vi "UpdateField.vi"   [LabVIEW 2025]
uses:
  ServerGlobalVariables.vi
types:
  T1 = typedef "FieldCell.ctl" = cluster{"Troops":u32, "Owner":i32, "Terrain":T2}
  T2 = typedef "TerrainEnum.ctl" = enum16{"Plain", "Mountain", "City", "General"}
  T3 = map{u32, cluster{"Name":string, "Team":u8, "Ready":bool, "Host":bool, "Alive":bool, "Color":u32, "Lands":set{cluster{"Row":u32, "Column":u32}}, "Army":u32}}
  T4 = cluster{"Name":string, "Team":u8, "Ready":bool, "Host":bool, "Alive":bool, "Color":u32, "Lands":set{cluster{"Row":u32, "Column":u32}}, "Army":u32}
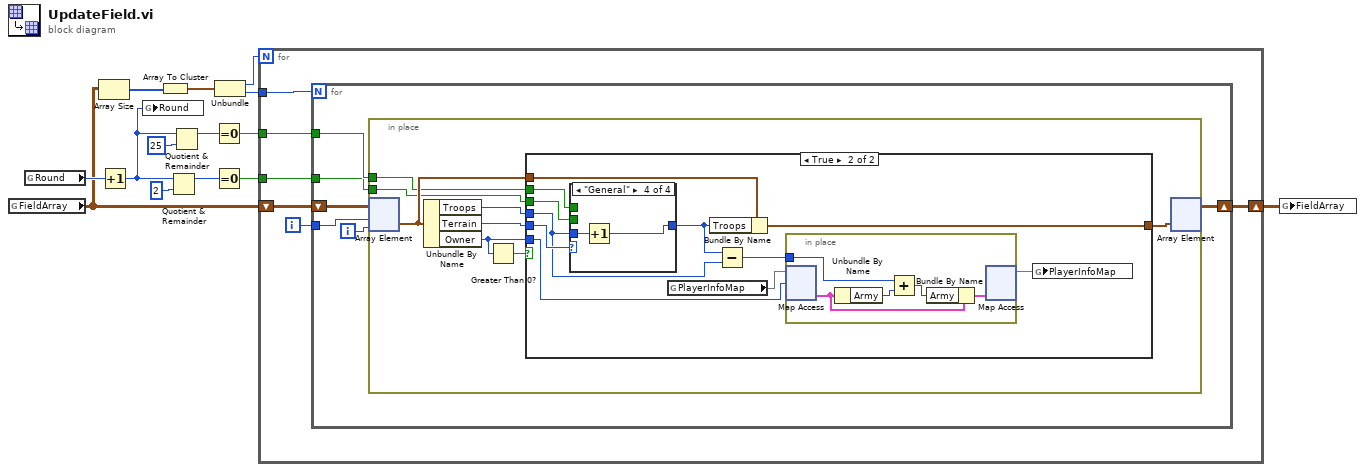
[diagram p0: block diagram]
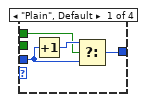
[diagram p3: hidden frame]
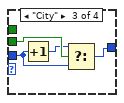
[diagram p5: hidden frame]
diagram:
  n1 = global read "ServerGlobalVariables.vi" "FieldArray"() -> (w8:T1[][])
  n2 = global read "ServerGlobalVariables.vi" "Round"() -> (w14:u32)
  n3 = Array Size(array=w8) -> (size(s)=w7:i32[])
  n4 = Increment(x=w14) -> (x+1=w11:u32)
  n5 = global write "ServerGlobalVariables.vi" "Round"(w11) -> ()
  n6 = Array To Cluster(array=w7) -> (cluster=w6:cluster{"[0]":i32, "[1]":i32})
  n7 = Quotient & Remainder(x=w11, y=u32 2) -> (x-y*floor(x/y)=w9:u32)  [unwired: 1 out]
  n8 = Quotient & Remainder(x=w11, y=u32 25) -> (x-y*floor(x/y)=w10:u32)  [unwired: 1 out]
  n9 = Equal To 0?(x=w10) -> (x = 0?=w2:bool)
  n10 = Equal To 0?(x=w9) -> (x = 0?=w1:bool)
  n11 = Unbundle(w6) -> ("[0]"=w5:i32, "[1]"=w4:i32)
  n12 = for {
    N: w5 -> [_]
    tunnel: w4 -> [w19]
    shift-right: [w17] -> w3
    shift-left: w8 -> [w20]
    tunnel: w2 -> [w16]
    tunnel: w1 -> [w15]
    i -> [w18]
    n13 = for {
      N: w19 -> [_]
      shift-right: [w23] -> w17
      shift-left: w20 -> [w24]
      tunnel: w18 -> [w26]
      tunnel: w16 -> [w22]
      tunnel: w15 -> [w21]
      i -> [w25]
      n14 = in-place {
        in-place-border: w22 -> [w31]
        in-place-border: w21 -> [w30]
        n15 = in-place-array #1(w24, w26, w25) -> (w33:T1)
        n16 = Unbundle By Name(w33) -> ("Troops"=w29:u32, "Terrain"=w34:T2, "Owner"=w28:i32)
        n17 = Greater Than 0?(x=w28) -> (x > 0?=w27:bool)
        n18 = case shown="True" w27 {
          tunnel: w34 -> [_ w46]
          tunnel: w33 -> [w35 w45]
          tunnel: [w35 w44] -> w32
          tunnel: w31 -> [_ w43]
          tunnel: w30 -> [_ w42]
          tunnel: w28 -> [_ w40]
          tunnel: w29 -> [_ w38]
          frame False {
          }
          frame True {
            n19 = case shown="\"General\"" w46 {
              tunnel: w38 -> [w54 w56 w58 w62]
              tunnel: [w53 w56 w59 w61] -> w39
              tunnel: w43 -> [w52 _ _ _]
              tunnel: w42 -> [_ _ w60 _]
              frame "Plain", Default {
                n20 = Increment(x=w54) -> (x+1=w55:u32)
                n21 = Select(t=w55, s=w52, f=w54) -> (s? t:f=w53:u32)
              }
              frame "Mountain" {
              }
              frame "City" {
                n22 = Increment(x=w58) -> (x+1=w57:u32)
                n23 = Select(t=w57, s=w60, f=w58) -> (s? t:f=w59:u32)
              }
              frame "General" {
                n24 = Increment(x=w62) -> (x+1=w61:u32)
              }
            }
            n25 = global read "ServerGlobalVariables.vi" "PlayerInfoMap"() -> (w41:T3)
            n26 = Bundle By Name(cluster=w45, "Troops"=w39) -> (w44:T1)
            n27 = Subtract(x=w39, y=w38) -> (x-y=w37:u32)
            n28 = in-place {
              in-place-border: w37 -> [w48]
              n29 = in-place-map #2(w41, w40) -> (w50:T4)  [unwired: 1 in, 1 out]
              n30 = Unbundle By Name(w50) -> ("Army"=w47:u32)
              n31 = Add(x=w48, y=w47) -> (x+y=w49:u32)
              n32 = Bundle By Name(cluster=w50, "Army"=w49) -> (w51:T4)
              n33 = in-place-map #2(w51) -> (w36:T3)  [unwired: 1 in, 2 out]
            }
            n34 = global write "ServerGlobalVariables.vi" "PlayerInfoMap"(w36) -> ()
          }
        }
        n35 = in-place-array #1(w32) -> (w23:T1[][])  [unwired: 2 out]
      }
    }
  }
  n36 = global write "ServerGlobalVariables.vi" "FieldArray"(w3) -> ()
